vi "I2C Number.vi"(4 "I2C in":refnum<class "I2C.lvclass">) -> (7 "I2C #":T1=-1)   [LabVIEW 2020, in "CTI.lvlib" / "I2C.lvclass"]
uses:
  I2C.lvclass
  I2C Number.ctl
  I2C.lvclass/I2C.ctl
  CTI.lvlib
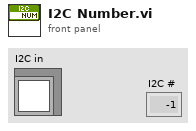
[diagram p1: front panel]
types:
  T1 = typedef "CTI.lvlib/I2C Number.ctl" = i8
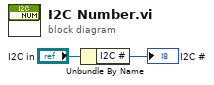
[diagram p0: block diagram]
diagram:
  n1 = Unbundle By Name("I2C in") -> ("I2C #"=→"I2C #":T1)
